vi "Append Copyright to Description.vi"(8 "Delimiter":string, 9 "Copyright Text":string, 11 "Description":string) -> (3 "Description out":string)   [LabVIEW 2020, in "VI Properties Editor.lvlib"]
doc: "Appends <B>Copyright Text</B> to <B>Description</B>."
uses:
  VI Properties Editor.lvlib
  <vilib>/Utility/error.llb/Trim Whitespace (string).vi
  <vilib>/Utility/error.llb/Trim Whitespace One-Sided.vi
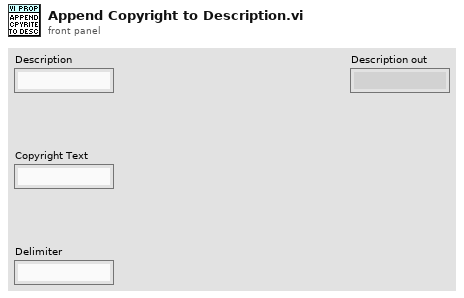
[diagram p1: front panel]
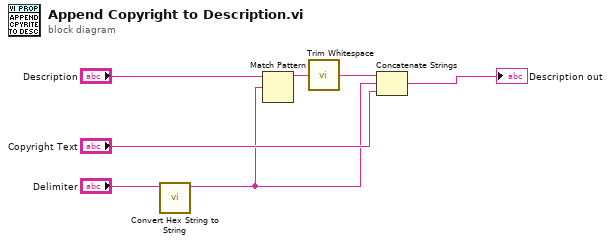
[diagram p0: block diagram]
diagram:
  n1 = call "Convert Hex String to String.vi"("Hex String"="Delimiter") -> ("String"=w1:string)  [unwired: 10 in]
  n2 = Match Pattern(string="Description", regular expression=w1) -> (before substring=w5:string)  [unwired: 1 in, 3 out]
  n3 = call-poly <vilib>:"Trim Whitespace.vi"("string"=w5) -> ("trimmed string"=w7:string)  [unwired: 1 in]
  n4 = Concatenate Strings(w7, w1, "Copyright Text") -> (→"Description out":string)
